vi "读取所有路计数器的原码值.vi"(8 "错误输入":errorcluster caption="错误输入（无错误）", 11 "设备句柄入":i32) -> (0 "错误输出":errorcluster, 1 "计数器的原码值":u32[](array[numeric]), 3 "设备句柄":i32=1)   [LabVIEW 2016]
uses:
  dll/em9636.dll
panel:
  in  "超时毫秒":i32=1000
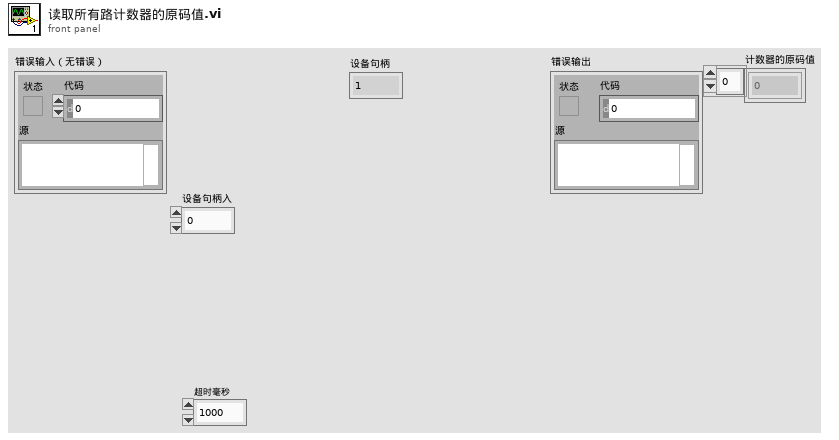
[diagram p1: front panel]
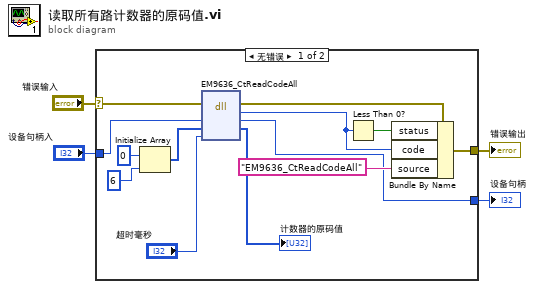
[diagram p0: block diagram]
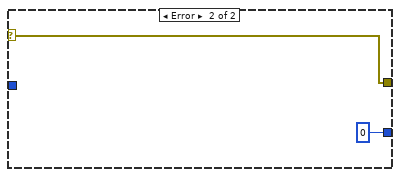
[diagram p2: hidden frame]
diagram:
  n1 = case shown="无错误" "错误输入" {
    selector: "错误输入" -> [w17 w19]
    tunnel: [w13 w19] -> w3
    tunnel: [w9 0 ("错误")] -> w2
    tunnel: "设备句柄入" -> [w11 _]
    frame No Error {
      n2 = Initialize Array(u32 0 ("元素"), 6 ("维数大小")) -> (w7:u32[])
      n3 = dll-call lib="PTH2kabs CUsers\nAdministratorDesktopEM9636*EM9636系列_demo_labview(调用DLL方式)dll\nem9636.dll" fn="EM9636_CtReadCodeAll"(error in=w17, "设备句柄"=w11, "ctCode"=w7, "超时毫秒"="超时毫秒") -> (error out=w15:errorcluster, "错误"=w12:i32, "设备句柄"=w9:i32, "ctCode"=→"计数器的原码值":u32[])  [unwired: 3 in, 1 out]
      n4 = Less Than 0?(x=w12) -> (x < 0?=w14:bool)
      n5 = Bundle By Name(cluster=w15, "status"=w14, "code"=w12, "source"="EM9636_CtReadCodeAll") -> (w13:errorcluster)
    }
    frame Error {
    }
  }
  "错误输出" <- w3
  "设备句柄" <- w2
